vi "Get Connections Dispatcher.vi"(6 "site":i32, 8 "error in":errorcluster, 9 "instrument":refnum<class "IInstrument.lvclass">, 10 "pin or relay names":string[](array[string]), 11 "session reservation in":refnum<class "Session Reservation.lvclass">) -> (0 "error out":errorcluster, 2 "connections":T1[](array[typedef]), 3 "session reservation out":refnum<class "Session Reservation.lvclass">)   [LabVIEW 2020, in "MeasurementLink Session Management.lvlib" / "Session Reservation.lvclass"]
uses:
  Session Reservation.lvclass
  Session Reservation.lvclass/Session Reservation.ctl
  IState/IState.lvclass
  Connection.ctl
  Connection with Session.ctl
  MeasurementLink Instrument/IInstrument/IInstrument.lvclass
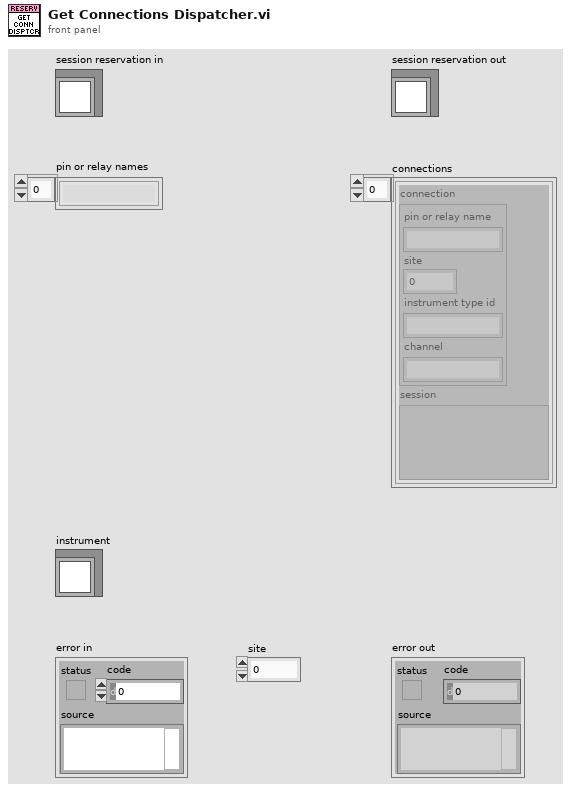
[diagram p1: front panel]
types:
  T1 = typedef "MeasurementLink Session Management.lvlib/Session Reservation.lvclass/Connection with Session.ctl" = cluster{"connection":T2, "session":variant}
  T2 = typedef "MeasurementLink Session Management.lvlib/Session Reservation.lvclass/Connection.ctl" = cluster{"pin or relay name":string, "site":i32, "instrument type id":string, "channel":string}
  T3 = typedef "MeasurementLink Session Management.lvlib/Session Reservation.lvclass/Data.ctl" = cluster{"session and driver infos":T4[], "pin or relay names":string[], "connection map":refnum<class "Connection Map.lvclass">, "pin map context":T8, "state":refnum<class "IState.lvclass">}
  T4 = typedef "MeasurementLink Session Management.lvlib/Session Reservation.lvclass/Session and Driver Info.ctl" = cluster{"session info":T5, "session":variant, "instrument":refnum<class "IInstrument.lvclass">}
  T5 = typedef "MeasurementLink Session Management Client.lvlib/ni_measurementlink_sessionmanagement_v1_SessionInformation.ctl" = cluster{"session":T6, "resource_name":string, "channel_list":string, "instrument_type_id":string, "session_exists":bool, "channel_mappings":T7[]}
  T6 = typedef "MeasurementLink Session Management Client.lvlib/nidevice_grpc_Session.ctl" = cluster{"name":string}
  T7 = typedef "MeasurementLink Session Management Client.lvlib/ni_measurementlink_sessionmanagement_v1_ChannelMapping.ctl" = cluster{"pin_or_relay_name":string, "site":i32, "channel":string}
  T8 = typedef "MeasurementLink Session Management Client.lvlib/ni_measurementlink_PinMapContext.ctl" = cluster{"pin_map_id":string, "sites":i32[]}
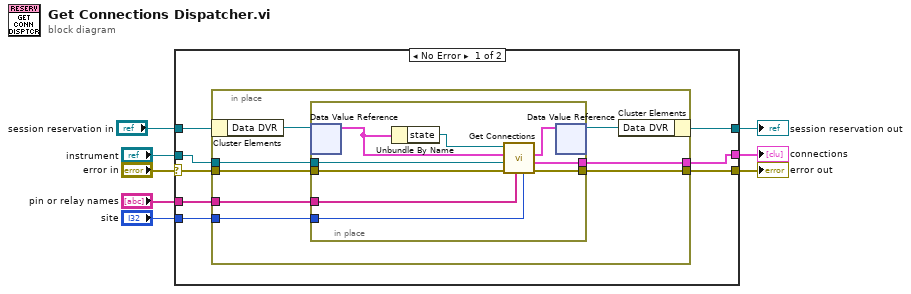
[diagram p0: block diagram]
diagram:
  n1 = case shown="No Error" "error in" {
    selector: "error in" -> [w13 w34]
    tunnel: "pin or relay names" -> [w12 _]
    tunnel: "site" -> [w11 _]
    tunnel: "instrument" -> [w14 _]
    tunnel: [w9 _] -> w4
    tunnel: "session reservation in" -> [w16 w35]
    tunnel: [w15 w35] -> w2
    tunnel: [w10 w34] -> w1
    frame No Error {
      n2 = in-place {
        in-place-border: w14 -> [w22]
        in-place-border: w13 -> [w21]
        in-place-border: w12 -> [w20]
        in-place-border: w11 -> [w19]
        in-place-border: [w18] -> w10
        in-place-border: [w17] -> w9
        n3 = in-place-cluster #1(w16) -> ("Data DVR"=w24:refnum<data-value>)
        n4 = in-place {
          in-place-border: w22 -> [w30]
          in-place-border: w21 -> [w29]
          in-place-border: w20 -> [w28]
          in-place-border: w19 -> [w27]
          in-place-border: [w26] -> w18
          in-place-border: [w25] -> w17
          n5 = in-place-dvr #2(w24) -> (w33:T3)  [unwired: 1 out]
          n6 = Unbundle By Name(w33) -> ("state"=w32:refnum<class "IState.lvclass">)
          n7 = call-dynamic "Get Connections.vi"("site"=w27, "pin or relay names"=w28, "error in"=w29, "instrument"=w30, "data in"=w33, "state in"=w32) -> ("error out"=w26:errorcluster, "connections"=w25:T1[], "data out"=w31:T3)  [unwired: 3 in]
          n8 = in-place-dvr #2(w31) -> (w23:refnum<data-value>)  [unwired: 1 out]
        }
        n9 = in-place-cluster #1("Data DVR"=w23) -> (w15:refnum<class "Session Reservation.lvclass">)
      }
    }
    frame Error {
    }
  }
  "error out" <- w1
  "connections" <- w4
  "session reservation out" <- w2
